vi "To JSON.vi"(8 "error in":errorcluster, 11 "PDO Communication Parameter in":refnum<class "PDO Communication Parameter.lvclass">) -> (0 "error out":errorcluster, 2 "<JSON>":string, 3 "PDO Communication Parameter out":refnum<class "PDO Communication Parameter.lvclass">)   [LabVIEW 2024, in "PDO Grid.lvlib" / "PDO Communication Parameter.lvclass"]
uses:
  PDO Communication Parameter.lvclass
  Access Type.ctl
  PDO Communication Parameter.lvclass/PDO Communication Parameter.ctl
  3d1835c6-3bd6-4528-a86e-98c144b88915.vi
  <vilib>/JDP Science/JSONtext/Variant to JSON Text.vi
  <vilib>/JDP Science/JSONtext/LVClass Serializer/JSONtext LVClass Serializer.lvclass
  Electronic Datasheet.lvlib
  <vilib>/JDP Science/JSONtext/JSONtext.lvlib
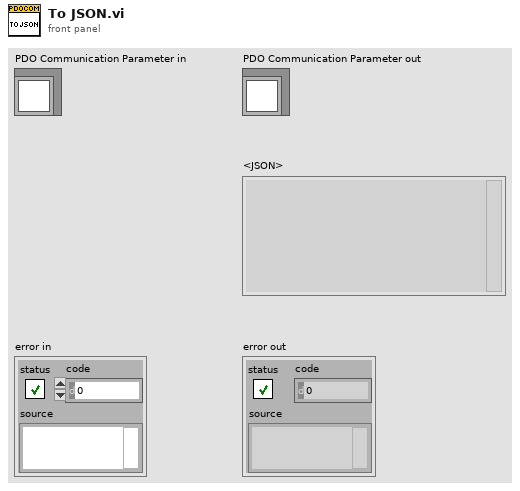
[diagram p1: front panel]
types:
  T1 = typedef "Electronic Datasheet.lvlib/Access Type.ctl" = enum16{"ro", "wo", "rw", "rwr", "rww", "const"}
  T2 = cluster{"Inhibit Time":u16, "Event-Timer":u16, "SYNC start value":u8, "COB-ID":u32, "OD Index":u16, "AccessType":T1, "Description":string}
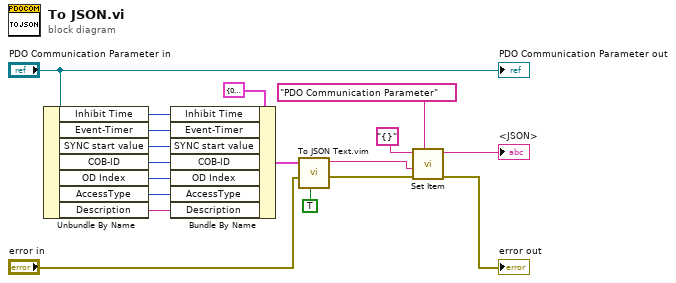
[diagram p0: block diagram]
diagram:
  n1 = Unbundle By Name("PDO Communication Parameter in") -> ("Inhibit Time"=w17:u16, "Event-Timer"=w16:u16, "SYNC start value"=w15:u8, "COB-ID"=w14:u32, "OD Index"=w13:u16, "AccessType"=w12:T1, "Description"=w11:string)
  n2 = Bundle By Name(cluster=T2 {"Inhibit Time"=0, "Event-Timer"=0, "SYNC start value"=0, "COB-ID"=0, "OD Index"=0, "AccessType"=enum."const", "Description"=""} ("Cluster of class private data"), "Inhibit Time"=w17, "Event-Timer"=w16, "SYNC start value"=w15, "COB-ID"=w14, "OD Index"=w13, "AccessType"=w12, "Description"=w11) -> (w9:T2)
  n3 = call "To JSON Text.vim"("Pretty Print?"=TRUE, "error in (no error)"="error in", "Anything"=w9) -> ("error out"=w4:errorcluster, "<JSON>"=w5:string)  [unwired: 7 in]
  n4 = call <vilib>:"Set Item.vi"("$Path or Item Name"="PDO Communication Parameter", "error in (no error)"=w4, "JSON to Insert"=w5, "JSON"="{}") -> ("error out"=→"error out":errorcluster, "<JSON>"=→"<JSON>":string)  [unwired: 4 in, 1 out]
  "PDO Communication Parameter out" <- "PDO Communication Parameter in"
